vi "Camera Focus Quality_Modified_24Jul21.vi"(7 "error in":errorcluster, 9 "stop":bool) -> (0 "error out":errorcluster, 1 "Final Result":bool, 2 "Pattern Presence":bool, 3 "Acquired Image":T1(plugin-control))   [LabVIEW 2018]
doc: "This VI demonstrates how to calculate the relative edge sharpness of an image to determine the best camera focus."
uses:
  <vilib>/vision/NI_Vision_Development_Module.lvlib
panel:
  out "Bottom_RH":bool
  out "RH_BOTTOM":string caption="Read String"
  out "Center_RH":bool
  out "RH_CENTER":string caption="Read String"
  out "Top_RH":bool
  out "RH_TOP":string caption="Read String"
  in  "Image Path":path=path "C:/images/img1.jpeg"
  out "y":sgl
  out "x":sgl
  out "Bottom":bool
  out "Bottom":string caption="Read String"
  out "Top":bool
  out "Top":string caption="Read String"
  out "Center":bool
  out "Center":string caption="Read String"
  out "Filtered Image":T1(plugin-control)
  out "Mean Value-Max":sgl format="%.2f"
  out "Waveform Chart":sgl(graph)
  in  "Filter Type":T2(ring)=enum."Differentiation"
  out "Current Mean Value":sgl format="%.2f"
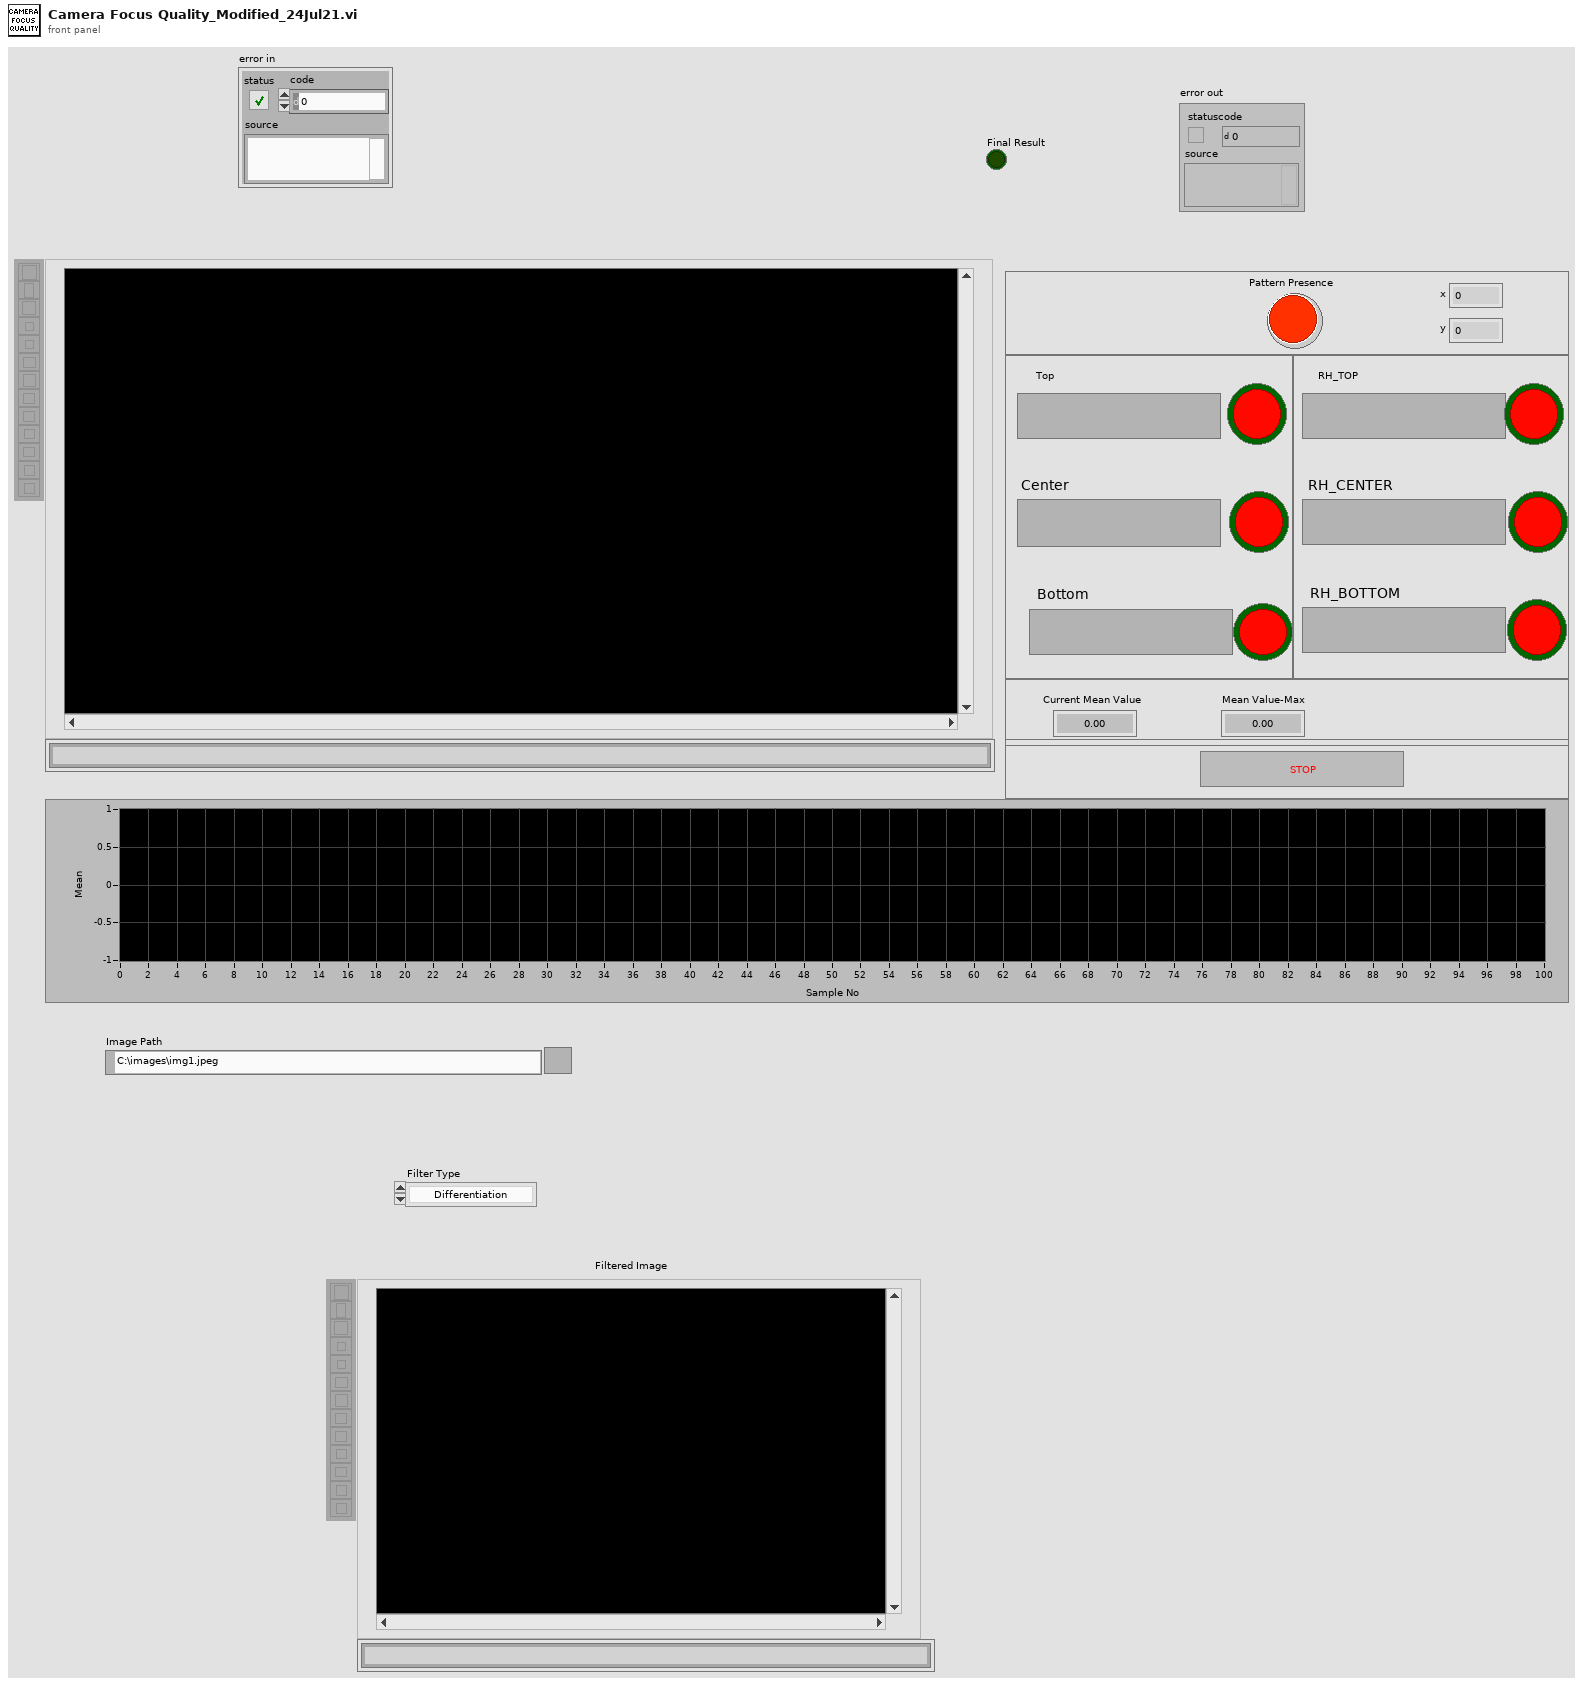
[diagram p1: front panel]
types:
  T1 = typedef "IMAQ Image.ctl" = refnum<image>
  T2 = enum16{"Convolution", "Differentiation", "Gradient", "Prewitt", "Roberts", "Sigma", "Sobel"}
  T3 = enum32{"Differentiation", "Gradient", "Prewitt", "Roberts", "Sigma", "Sobel"}
  T4 = typedef "Image Type" = u32
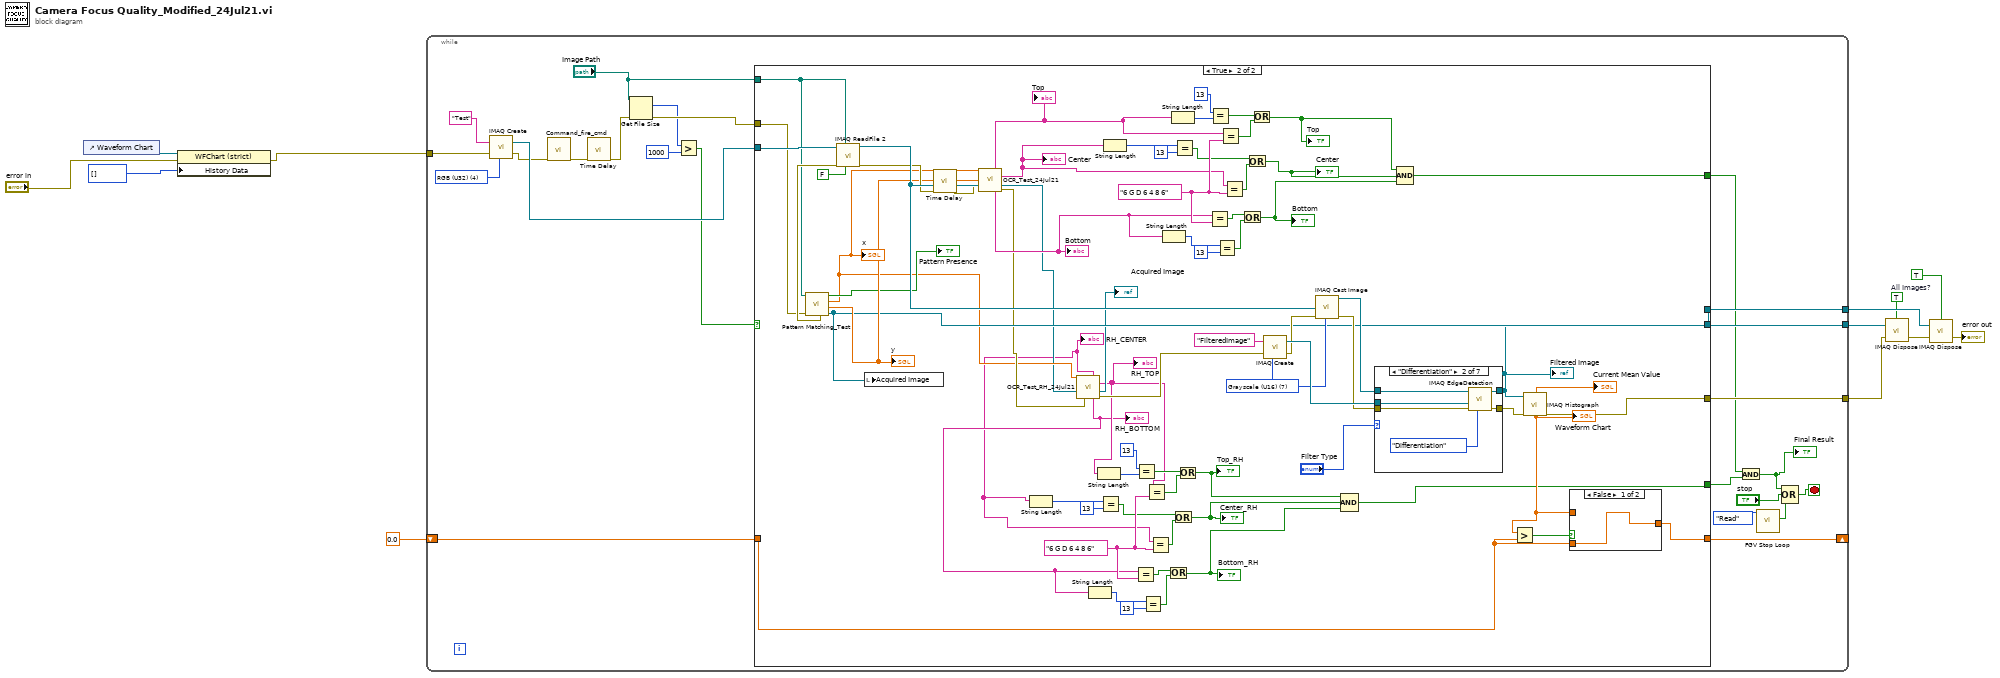
[diagram p0: block diagram]
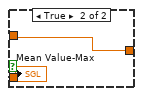
[diagram p3: hidden frame]
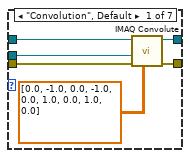
[diagram p4: hidden frame]
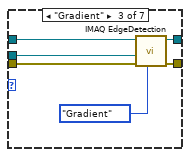
[diagram p5: hidden frame]
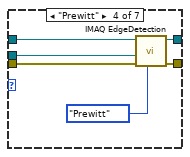
[diagram p6: hidden frame]
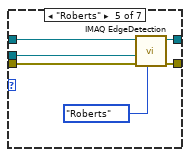
[diagram p7: hidden frame]
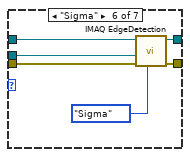
[diagram p8: hidden frame]
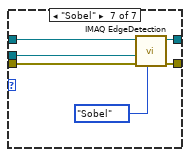
[diagram p9: hidden frame]
diagram:
  w6 = TRUE  # All Images?
  n1 = control-ref of="Waveform Chart"() -> (w11:refnum<vi>)
  n2 = property on="Property Node" class="WFChart (strict)"(reference=w11, error in="error in", "History Data"=u32[] []) -> (error out=w3:errorcluster)  [unwired: 1 out]
  n3 = while {
    shift-right: [w36] -> _
    shift-left: sgl 0.0 ("Mean Value - Max") -> [w35]
    tunnel: [w34] -> w7
    tunnel: [w33] -> w5
    tunnel: [w32] -> w4
    tunnel: w3 -> [w31]
    stop <- w15 stop-if-true
    w25 = T4 4 items=["Grayscale (U8)", "Grayscale (I16)", "Grayscale (SGL)", "Complex (CSG)", "RGB (U32)", "HSL (U32)", "RGB (U64)", "Grayscale (U16)"] ("Image Type")
    n4 = call "IMAQ Create"("Image Name"="Test", "Image Type"=w25, "error in (no error)"=w31) -> ("New Image"=w30:T1, "error out"=w24:errorcluster)  [unwired: 2 in]
    n5 = call "Command_fire_cmd.vi"("error in"=w24) -> ("error out"=w23:errorcluster)  [unwired: 6 in, 2 out]
    n6 = call "Time Delay"("error in (no error)"=w23) -> ("error out"=w27:errorcluster)  [unwired: 10 in]
    n7 = Get File Size(file="Image Path", error in=w27) -> (size (in bytes)=w22:i64, 0:w28:errorcluster)  [unwired: 1 out]
    n8 = Greater?(x=w22, y=i64 1000) -> (0:w20:bool)
    n9 = case shown="True" w20 {
      tunnel: [w37 w101] -> w36
      tunnel: w35 -> [w37 w97]
      tunnel: [_ w74] -> w34
      tunnel: [_ w73] -> w33
      tunnel: [w38 w72] -> w32
      tunnel: w30 -> [_ w70]
      tunnel: "Image Path" -> [_ w69]
      tunnel: w28 -> [w38 w68]
      tunnel: [_ w40] -> w18
      tunnel: [_ w39] -> w19
      frame False {
      }
      frame True {
        w62 = "6 G D 6 4 8 6" ("y")
        w96 = "6 G D 6 4 8 6" ("y")
        w106 = T4 7 items=["Grayscale (U8)", "Grayscale (I16)", "Grayscale (SGL)", "Complex (CSG)", "RGB (U32)", "HSL (U32)", "RGB (U64)", "Grayscale (U16)"] ("Image Type")
        n10 = call "Pattern Matching_Test.vi"("error in (no error)"=w68, "File Path"=w69) -> ("Image out"=w74:T1, "y"=w77:sgl, "x"=w65:sgl, "Pattern Presence"=→"Pattern Presence":bool, "error out"=w71:errorcluster)  [unwired: 5 in]
        "x" <- w65
        "y" <- w77
        n11 = call "IMAQ ReadFile 2"("Use File Path Image Type"=FALSE, "File Path"=w69, "error in (no error)"=w71, "Image"=w70) -> ("error out"=w93:errorcluster, "Image Out"=w94:T1)  [unwired: 3 in, 3 out]
        n12 = local write "Acquired Image"(w74) -> ()
        n13 = call "Time Delay"("error in (no error)"=w93) -> ("error out"=w76:errorcluster)  [unwired: 10 in]
        n14 = call "OCR_Test_24Jul21.vi"("x"=w65, "y"=w77, "Image in"=w94, "error in (no error)"=w76) -> ("Read Top"=w92:string, "Read Center"=w91:string, "Image"=w64:T1, "Read bottom"=w90:string, "error out"=w67:errorcluster)  [unwired: 7 in]
        "Center" <- w91
        "Top" <- w92
        "Bottom" <- w90
        n15 = call "OCR_Test_RH_24Jul21.vi"(0:w65, "Image in"=w64, "error in (no error)"=w67) -> ("Read Center"=w47:string, "Read Top"=w49:string, "Image"=→"Acquired Image":T1, "Read bottom"=w48:string, "error out"=w66:errorcluster)  [unwired: 7 in, 1 out]
        "RH_TOP" <- w49
        "RH_CENTER" <- w47
        "RH_BOTTOM" <- w48
        n16 = String Length(string=w47) -> (length=w57:i32)
        n17 = String Length(string=w48) -> (length=w59:i32)
        n18 = String Length(string=w49) -> (length=w61:i32)
        n19 = Equal?(x=w57, y=13) -> (x = y?=w53:bool)
        n20 = String Length(string=w91) -> (length=w85:i32)
        n21 = Equal?(x=w48, y=w62) -> (x = y?=w51:bool)
        n22 = Equal?(x=13, y=w61) -> (x = y?=w54:bool)
        n23 = Equal?(x=w59, y=13) -> (x = y?=w50:bool)
        n24 = Equal?(x=w49, y=w62) -> (x = y?=w55:bool)
        n25 = Equal?(x=w47, y=w62) -> (x = y?=w52:bool)
        n26 = String Length(string=w90) -> (length=w87:i32)
        n27 = Or(x=w51, y=w50) -> (x .or. y?=w41:bool)
        "Bottom_RH" <- w41
        n28 = String Length(string=w92) -> (length=w89:i32)
        n29 = Or(x=w53, y=w52) -> (x .or. y?=w42:bool)
        "Center_RH" <- w42
        n30 = Equal?(x=w85, y=13) -> (x = y?=w81:bool)
        n31 = Or(x=w54, y=w55) -> (x .or. y?=w43:bool)
        "Top_RH" <- w43
        n32 = Equal?(x=w90, y=w96) -> (x = y?=w79:bool)
        n33 = Equal?(x=13, y=w89) -> (x = y?=w82:bool)
        n34 = Equal?(x=w87, y=13) -> (x = y?=w78:bool)
        n35 = Equal?(x=w92, y=w96) -> (x = y?=w83:bool)
        n36 = Equal?(x=w91, y=w96) -> (x = y?=w80:bool)
        n37 = Or(x=w79, y=w78) -> (x .or. y?=w44:bool)
        "Bottom" <- w44
        n38 = Or(x=w81, y=w80) -> (x .or. y?=w45:bool)
        "Center" <- w45
        n39 = Or(x=w82, y=w83) -> (x .or. y?=w46:bool)
        "Top" <- w46
        n40 = call "IMAQ Create"("Image Name"="FilteredImage", "Image Type"=w106, "error in (no error)"=w66) -> ("New Image"=w107:T1, "error out"=w105:errorcluster)  [unwired: 2 in]
        n41 = call "IMAQ Cast Image"("Image Type"=w106, "error in (no error)"=w105, "Image Src"=w94) -> ("error out"=w102:errorcluster, "Image Dst Out"=w98:T1)  [unwired: 7 in]
        n42 = Compound Arithmetic op=AND(w43, w42, w41) -> (w40:bool)
        n43 = case shown="\"Differentiation\"" "Filter Type" {
          tunnel: w98 -> [w115 w121 w127 w133 w139 w145 w151]
          tunnel: w102 -> [w114 w120 w126 w132 w138 w144 w150]
          tunnel: w107 -> [w113 w122 w128 w134 w140 w146 w152]
          tunnel: [w112 w117 w123 w129 w135 w141 w147] -> w104
          tunnel: [w111 w118 w124 w130 w136 w142 w148] -> w73
          frame "Convolution", Default {
            n44 = call "IMAQ Convolute"("Kernel"=sgl[][] [[0.0, -1.0, 0.0], [-1.0, 0.0, 1.0], [0.0, 1.0, 0.0]], "error in (no error)"=w114, "Image Dst"=w113, "Image Src"=w115) -> ("error out"=w112:errorcluster, "Image Dst Out"=w111:T1)  [unwired: 6 in]
          }
          frame "Differentiation" {
            n45 = call "IMAQ EdgeDetection"("Method"=T3."Differentiation", "error in (no error)"=w120, "Image Dst"=w122, "Image Src"=w121) -> ("error out"=w117:errorcluster, "Image Dst Out"=w118:T1)  [unwired: 6 in]
          }
          frame "Gradient" {
            n46 = call "IMAQ EdgeDetection"("Method"=T3."Gradient", "error in (no error)"=w126, "Image Dst"=w128, "Image Src"=w127) -> ("error out"=w123:errorcluster, "Image Dst Out"=w124:T1)  [unwired: 6 in]
          }
          frame "Prewitt" {
            n47 = call "IMAQ EdgeDetection"("Method"=T3."Prewitt", "error in (no error)"=w132, "Image Dst"=w134, "Image Src"=w133) -> ("error out"=w129:errorcluster, "Image Dst Out"=w130:T1)  [unwired: 6 in]
          }
          frame "Roberts" {
            n48 = call "IMAQ EdgeDetection"("Method"=T3."Roberts", "error in (no error)"=w138, "Image Dst"=w140, "Image Src"=w139) -> ("error out"=w135:errorcluster, "Image Dst Out"=w136:T1)  [unwired: 6 in]
          }
          frame "Sigma" {
            n49 = call "IMAQ EdgeDetection"("Method"=T3."Sigma", "error in (no error)"=w144, "Image Dst"=w146, "Image Src"=w145) -> ("error out"=w141:errorcluster, "Image Dst Out"=w142:T1)  [unwired: 6 in]
          }
          frame "Sobel" {
            n50 = call "IMAQ EdgeDetection"("Method"=T3."Sobel", "error in (no error)"=w150, "Image Dst"=w152, "Image Src"=w151) -> ("error out"=w147:errorcluster, "Image Dst Out"=w148:T1)  [unwired: 6 in]
          }
        }
        "Filtered Image" <- w73
        n51 = Compound Arithmetic op=AND(w46, w45, w44) -> (w39:bool)
        n52 = call "IMAQ Histograph"("error in (no error)"=w104, "Image"=w73) -> ("error out"=w72:errorcluster, "Mean Value"=w100:sgl)  [unwired: 6 in, 2 out]
        "Current Mean Value" <- w100
        "Waveform Chart" <- w100
        n53 = Greater?(x=w100, y=w97) -> (0:w99:bool)
        n54 = case shown="False" w99 {
          tunnel: w100 -> [_ w110]
          tunnel: [w109 w110] -> w101
          tunnel: w97 -> [w109 _]
          frame False {
          }
          frame True {
            "Mean Value-Max" <- w110
          }
        }
      }
    }
    n55 = And(x=w19, y=w18) -> (x .and. y?=w17:bool)
    "Final Result" <- w17
    n56 = call "FGV Stop Loop.vi"("Action"=enum16{"Initialize", "Read", "Write"}."Read") -> ("Out"=w14:bool)  [unwired: 9 in, 1 out]
    n57 = Compound Arithmetic op=OR(w17, "stop", w14) -> (w15:bool)
  }
  n58 = call "IMAQ Dispose"("All Images? (No)"=w6, "Image"=w5, "error in (no error)"=w4) -> ("error out"=w9:errorcluster)  [unwired: 3 in]
  n59 = call "IMAQ Dispose"("All Images? (No)"=TRUE, "Image"=w7, "error in (no error)"=w9) -> ("error out"=→"error out":errorcluster)  [unwired: 3 in]
